vi "HackyNICard.vi"() -> ()   [LabVIEW 2013]
uses:
  <vilib>/DAQmx/write.llb/DAQmx Write (Analog 2D DBL NChan NSamp).vi
  <vilib>/DAQmx/configure/timing.llb/DAQmx Timing (Sample Clock).vi
  <vilib>/DAQmx/miscellaneous.llb/DAQmx Fill In Error Info.vi
panel:
  in  "stop":bool
  out "error out":errorcluster
  out "Array":dbl[][](array[numeric])
  in  "Clock line":tag
  in  "Steps":i32
  in  "Ramp Values":T1(array[cluster])
  in  "Static Values":cluster{"Channel":refnum<k21>, "Value":dbl}[](array[cluster])
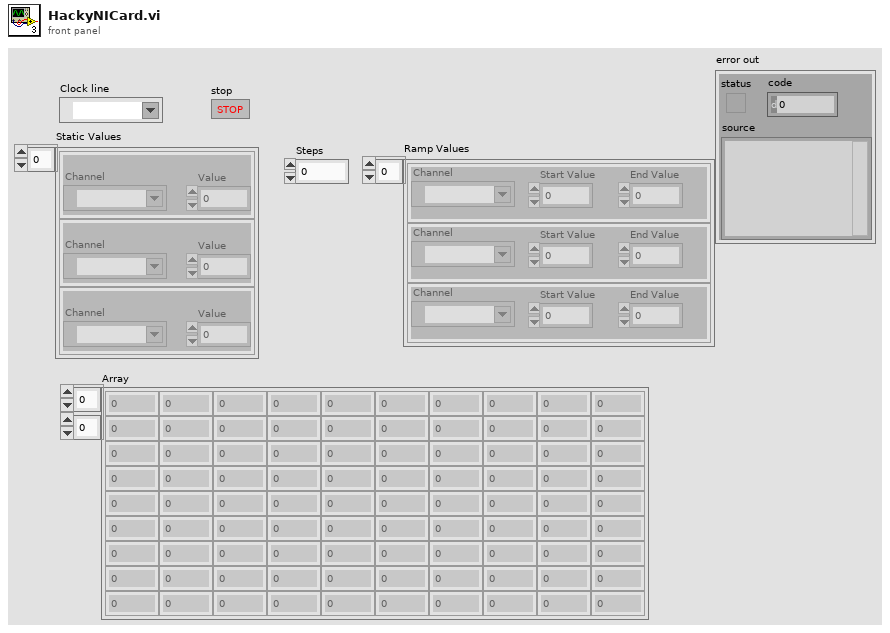
[diagram p1: front panel]
types:
  T1 = cluster{"Channel":refnum<k21>, "Start Value":dbl, "End Value":dbl}[]
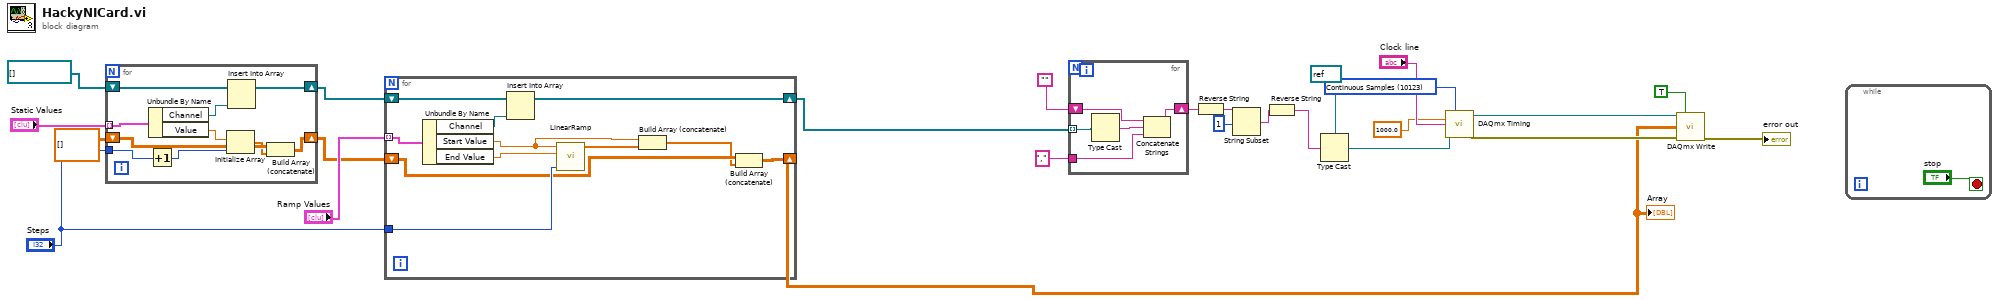
[diagram p0: block diagram]
diagram:
  w10 = 10123 items=["Finite Samples"=10178, "Continuous Samples"=10123, "Hardware Timed Single Point"=12522] ("sample mode")
  n1 = for {
    tunnel: "Static Values" -> [w35] mode=indexing
    shift-right: [w32] -> w21
    shift-left: refnum<k21>[] [] ("array") -> [w33]
    tunnel: "Steps" -> [w27]
    shift-right: [w29] -> w7
    shift-left: dbl[][] [] -> [w30]
    n2 = Unbundle By Name(w35) -> ("Channel"=w34:refnum<k21>, "Value"=w31:dbl)
    n3 = Increment(x=w27) -> (x+1=w26:i32)
    n4 = Initialize Array(w31, w26) -> (w28:dbl[])
    n5 = Insert Into Array(array=w33, new element=w34) -> (w32:refnum<k21>[])  [unwired: 1 in]
    n6 = Build Array (concatenate)(w30, w28) -> (w29:dbl[][])
  }
  n7 = for {
    tunnel: "Ramp Values" -> [w46] mode=indexing
    shift-right: [w43] -> w12
    shift-left: w21 -> [w44]
    shift-right: [w39] -> w5
    shift-left: w7 -> [w40]
    tunnel: "Steps" -> [w41]
    n8 = Unbundle By Name(w46) -> ("Channel"=w45:refnum<k21>, "Start Value"=w38:dbl, "End Value"=w42:dbl)
    n9 = Insert Into Array(array=w44, new element=w45) -> (w43:refnum<k21>[])  [unwired: 1 in]
    n10 = call "LinearRamp.vi"("Steps"=w41, "End Value"=w42, "Start Value"=w38) -> ("Ramp Out"=w37:dbl[])  [unwired: 8 in]
    n11 = Build Array (concatenate)(w38, w37) -> (w36:dbl[])
    n12 = Build Array (concatenate)(w40, w36) -> (w39:dbl[][])
  }
  "Array" <- w5
  n13 = for {
    tunnel: w12 -> [w51] mode=indexing
    shift-right: [w48] -> w18
    shift-left: "" -> [w50]
    tunnel: "," -> [w49]
    n14 = Type Cast(x=w51) -> (*(type *) &x=w47:string)  [unwired: 1 in]
    n15 = Concatenate Strings(w50, w47, w49) -> (w48:string)
  }
  n16 = Reverse String(1:w18) -> (0:w17:string)
  n17 = String Subset(string=w17, offset (0)=1) -> (substring=w16:string)  [unwired: 1 in]
  n18 = Reverse String(1:w16) -> (0:w14:string)
  n19 = Type Cast(type=refnum<k21> refnum ("DAQmx Global Channel"), x=w14) -> (*(type *) &x=w11:refnum<k21>)
  n20 = call-poly <vilib>:"DAQmx Timing.vi"("task/channels in"=w11, "sample mode"=w10, "rate"=1000.0, "source"="Clock line") -> ("task out"=w9:refnum<k21>, "error out"=w8:errorcluster)  [unwired: 10 in]
  n21 = call-poly <vilib>:"DAQmx Write.vi"("task/channels in"=w9, "auto start"=TRUE, "data"=w5, "error in"=w8) -> ("error out"=→"error out":errorcluster)  [unwired: 9 in, 2 out]
  n22 = while {
    stop <- "stop" stop-if-true
  }
